vi "pid-sim-motor.vi"(6 "Use Noise":bool, 9 "Cycle Time":dbl, 10 "CO-ControlOutput":dbl) -> (3 "Motor Speed":dbl)   [LabVIEW 2019]
uses:
  <vilib>/addons/control/pid/pid.llb/PID Lead-Lag (DBL).vi
  <vilib>/addons/control/pid/NI_PID_pid.lvlib
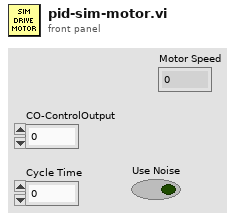
[diagram p1: front panel]
types:
  T1 = cluster{"gain":dbl, "lag time":dbl, "lead time":dbl}
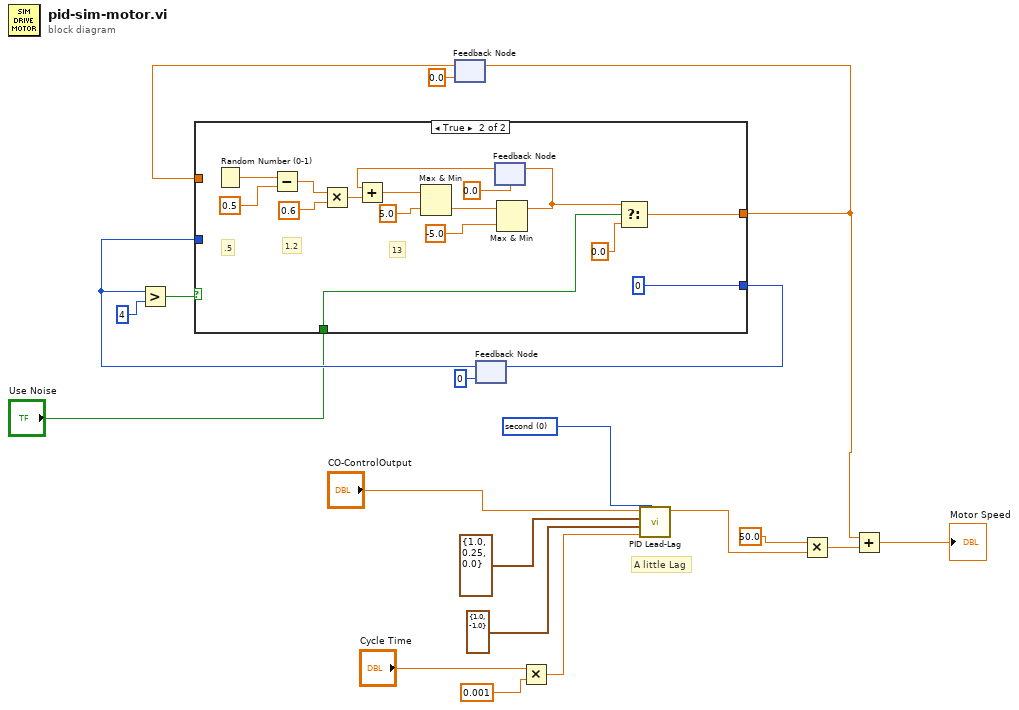
[diagram p0: block diagram]
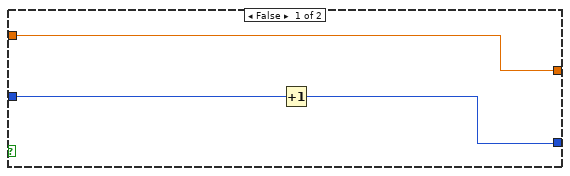
[diagram p2: hidden frame]
diagram:
  w20 = u16 0 items=["second", "minute"] ("time unit")
  # "A little Lag"
  n1 = feedback #1(0.0 ("f")) -> (w2:dbl)
  n2 = feedback #2(0) -> (w5:i32)
  n3 = Greater?(x=w5, y=4) -> (0:w7:bool)
  n4 = case shown="True" w7 {
    tunnel: [w22 0] -> w9
    tunnel: w5 -> [w23 _]
    tunnel: [w21 w25] -> w4
    tunnel: w2 -> [w21 _]
    tunnel: "Use Noise" -> [_ w24]
    frame False {
      n5 = Increment(x=w23) -> (x+1=w22:i32)
    }
    frame True {
      # "13"
      # "1.2"
      # ".5"
      n6 = Random Number (0-1)() -> (number: 0 to 1=w28:dbl)
      n7 = Subtract(x=w28, y=0.5) -> (x-y=w32:dbl)
      n8 = Multiply(x=w32, y=0.6) -> (x*y=w31:dbl)
      n9 = feedback #3(0.0) -> (w34:dbl)
      n10 = Add(x=w34, y=w31) -> (x+y=w38:dbl)
      n11 = Max & Min(x=w38, y=5.0) -> (min(x,y)=w37:dbl)  [unwired: 1 out]
      n12 = Max & Min(x=w37, y=-5.0) -> (max(x,y)=w29:dbl)  [unwired: 1 out]
      n13 = feedback-in #3(w29) -> ()
      n14 = Select(t=w29, s=w24, f=0.0) -> (s? t:f=w25:dbl)
    }
  }
  n15 = feedback-in #1(w4) -> ()
  n16 = feedback-in #2(w9) -> ()
  n17 = Multiply(x="Cycle Time", y=0.001) -> (x*y=w11:dbl)
  n18 = call-poly <vilib>:"PID Lead-Lag.vi"("time unit"=w20, "dt (s)"=w11, "output range"=cluster{"output high":dbl, "output low":dbl} {"output high"=1.0, "output low"=-1.0}, "tuning parameters"=T1 {"gain"=1.0, "lag time"=0.25, "lead time"=0.0}, "input"="CO-ControlOutput") -> ("output"=w10:dbl)  [unwired: 3 in, 1 out]
  n19 = Multiply(x=50.0, y=w10) -> (x*y=w12:dbl)
  n20 = Add(x=w4, y=w12) -> (x+y=→"Motor Speed":dbl)
